vi "Value to float32 string.vi"(1 "Value":dbl) -> (0 "Float32 str (Little Endian)":string)   [LabVIEW 2015]
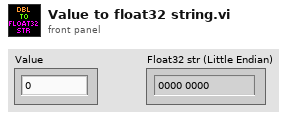
[diagram p1: front panel]
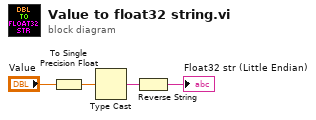
[diagram p0: block diagram]
diagram:
  n1 = To Single Precision Float(number="Value") -> (single precision float=w3:sgl)
  n2 = Type Cast(x=w3) -> (*(type *) &x=w4:string)  [unwired: 1 in]
  n3 = Reverse String(1:w4) -> (0:→"Float32 str (Little Endian)":string)
